vi "Cleanup.vi"(8 "error in (no error)":errorcluster, 11 "Mixer in":refnum<class "Mixer.lvclass">) -> (0 "error out":errorcluster, 3 "Mixer out":refnum<class "Mixer.lvclass">)   [LabVIEW 2018, in "Mixer.lvclass"]
uses:
  Mixer.lvclass
  Mixer.lvclass/Mixer.ctl
  Channel/Channel.lvclass
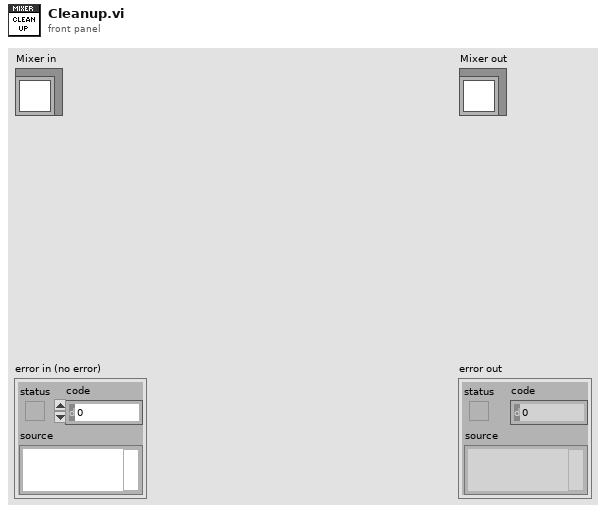
[diagram p1: front panel]
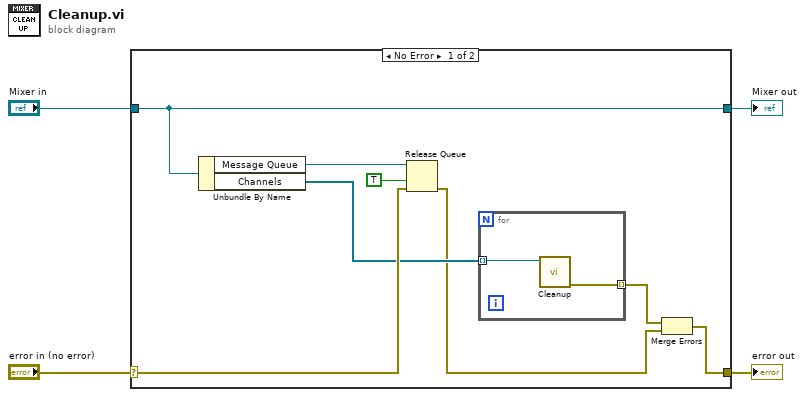
[diagram p0: block diagram]
diagram:
  n1 = case shown="No Error" "error in (no error)" {
    selector: "error in (no error)" -> [w10 w16]
    tunnel: [w5 w16] -> w3
    tunnel: [w12 w15] -> w1
    tunnel: "Mixer in" -> [w12 w15]
    frame No Error {
      n2 = Unbundle By Name(w12) -> ("Message Queue"=w11:refnum<queue>, "Channels"=w8:refnum<class "Channel.lvclass">[])
      n3 = Release Queue(queue=w11, force destroy? (F)=TRUE, error in (no error)=w10) -> (error out=w6:errorcluster)  [unwired: 2 out]
      n4 = for {
        tunnel: w8 -> [w14] mode=indexing
        tunnel: [w13] -> w7 mode=indexing
        n5 = call "Cleanup.vi"("Channel in"=w14) -> ("error out"=w13:errorcluster)  [unwired: 10 in]
      }
      n6 = Merge Errors(w7, w6) -> (w5:errorcluster)
    }
    frame Error {
    }
  }
  "error out" <- w3
  "Mixer out" <- w1
